vi "Photon Counter Control Panel.vi"(8 "error in (no error)":errorcluster) -> (0 "error out":errorcluster)   [LabVIEW 2015]
uses:
  Public/Typedefs/Gate Mode.ctl
  Public/Typedefs/Discriminator Output.ctl
  <vilib>/express/express shared/transition.llb/Dynamic To Waveform Array.vi
  <vilib>/express/express signal manip/GetorSetDDTAttributes/Set DDT Attributes/SetT0.vi
  <vilib>/express/express shared/transition.llb/Waveform Array To Dynamic.vi
  <vilib>/express/express signal manip/GetorSetDDTAttributes/Set DDT Attributes/Set DDT Properties.xnode
  SR400.lvlib
panel:
  in  "Monitor":bool
  in  "Start Scan":bool caption="Start Monitored Scan"
  in  "Stop Scan":bool
  out "Counter B":dbl(graph)=996.0
  out "Counter A":dbl(graph)=944.0
  out "Scan Start Time":timestamp=timestamp(3611338511.309165 s since 1904-01-01)
  out "Counter A":dbl(graph)=5052.0
  out "Counter B":dbl(graph)=5104.0
  in  "Read Buffer Data":bool
  out "Scan Done":bool
  out "Data Ready":bool
  in  "Query Status Byte":bool
  out "Scan Start Time":timestamp=timestamp(3611333596.390047 s since 1904-01-01)
  out "Filename Out":path=path "C:/Users/physics/Desktop/test_1.xlsx"
  in  "GPIB Address":i32=23 min=0 max=30 step=1
  in  "Stop Unmonitored Scan":bool
  in  "Disc A Mode":T1
  in  "Disc B Mode":T1
  in  "Disc B Slope":enum16{"Rise", "Fall"}(ring)
  in  "Disc A Slope":enum16{"Rise", "Fall"}(ring)
  in  "Trigger Slope":enum16{"Rise", "Fall"}(ring)
  in  "Set Gate Widths":bool
  in  "Set Gate Mode":bool
  out "Actual":dbl[unit]=0.5 caption="Current Dwell Time"
  in  "Target":dbl[unit]=0.5 caption="Dwell Time Target" min=0.0 max=60.0 step=0.5 format="%#_1g"
  in  "Set Dwell Time":bool
  in  "Target":i32=10 caption="Number of Periods Target" min=0 max=2000 step=1
  out "Actual":dbl=10.0 caption="Number of Periods Current"
  in  "Set # Periods":bool
  in  "Scan End Mode":enum16{"Stop", "Start"}(ring)
  in  "Disc B Lvl":dbl=-0.012 format="%#_13g"
  in  "Disc A Lvl":dbl=-0.012 format="%#_13g"
  in  "Display Mode":enum16{"Continuous", "Hold"}(ring)
  in  "Initialize":bool
  in  "Internal / External":bool
  in  "Set Count Time":bool
  in  "Counter B Input":enum16{"10 MHz", "INPUT 1", "INPUT 2", "TRIG"}(ring)=enum."INPUT 1"
  in  "Counter A Input":enum16{"10 MHz", "INPUT 1", "INPUT 2", "TRIG"}(ring)=enum."INPUT 1"
  in  "Count Mode":T2(ring)
  in  "Trigger Level":dbl=1.25 format="%#_13g"
  in  "VISA Resource Name":refnum<visa-resource-name>="GPIB0::23::INSTR"
  in  "Photon Counter SR 400":T3={"Mode"=0, "Count Time"=1.0, "Trigger Frequency"=10000000.0, "Trigger External?"=FALSE, "Gate A Mode"=0, "Gate A Width"=5e-09, "Gate A Delay"=5e-09, "Gate B Mode"=0, "Gate B Width"=5e-09, "Gate B Delay"=5e-09} {"Mode" items=["A,B For T Preset", "A-B For T Preset", "A+B For T Preset", "A For B Preset"]; "Gate A Mode" items=["CW", "Fixed"]; "Gate B Mode" items=["CW", "Fixed"]}
  out "Update visible/hidden":bool
  out "Actual":T4
  out "Actual":T4
  in  "stop":bool
  in  "Read to\nControl":bool
  in  "Read":bool
  out "Actual":dbl=5.0
  out "Actual":dbl=5.0
  in  "Target":dbl=5.0 caption="Gate A Width Percent Target"
  in  "Target":dbl=5.0 caption="Gate A Percent Target"
  in  "Gate Width: Time / Percent":bool caption="Time/Percent"
  in  "Start / Middle":bool
  in  "Target":T4 caption="Gate B Mode Target"
  in  "Target":T4 caption="Gate A Mode Target"
  out "Actual":dbl[unit]=10000000.0 caption="Trigger Freq"
  in  "Target":dbl[unit]=10000000.0 caption="Trigger Freq. Target"
  in  "Set Time & Freq.":bool
  in  "# Triggers vs Freq/Time":bool=TRUE
  out "Actual":dbl=10000000.0 caption="External Trigger # Cycles Current" format="%^#_6g"
  in  "Target":dbl=10000000.0 format="%^#_6g"
  in  "Set # of Triggers":bool
  in  "Target":dbl[unit]=5e-09 caption="Gate B Width Target"
  in  "Target":dbl[unit]=5e-09 caption="Gate A Width Target"
  out "Actual":dbl[unit]=5e-09 format="%^#_6g"
  out "Actual":dbl[unit]=5e-09 format="%^#_6g"
  out "Actual":dbl[unit]=5e-09
  out "Actual":dbl[unit]=5e-09
  in  "Target":dbl[unit]=5e-09
  in  "Target":dbl[unit]=5e-09 caption="Gate A Delay Target"
  in  "Set Gate Delays":bool
  in  "Start Unmonitored Scan":bool
  in  "Target":dbl[unit]=1.0 caption="Count Time Target" min=0.0 step=0.5 format="%#_1f"
  out "Actual":dbl[unit]=1.0 caption="Count Time Current" min=0.0 max=10000.0 step=1.0 format="%#_7g"
  # "Gates"
  # "Setup"
  # "Acquisition"
  # "Gate B Mode"
  # "Gate A Mode"
  # "# of Periods"
  # "Count Time"
  # "Gate A Width"
  # "Gate B Width"
  # "Dwell Time"
  # "Gate A Delay"
  # "Gate B Delay"
  # "Set values and initialize.\n\nSettings you can \"live\" update w/o initialization:\n        All Gate Params\n        Count Time (Only largest sig digit used)\n        Dwell Time (Only largest sig digit used)\n        External Trigger\n        # Periods\n\nSettings without a \"Set _____\" button need to be changed by initialization.\n\nAll variables are initialized, but \"live\" params do not show current value until you press the set button for that parameter.\n\n\"Read\" sets the \"Current\" indicators to what the hardware has set.\n\n\"Read to Control\" sets the \"Setpoint\" controls to the values from \"Read\""
  # "Discriminator/Trigger"
  # "Do not save data until after the scan is done or stopped.\n\nMonitored data may be erroneous due to communication delay\n\nTimestamps are relative to saving the data, not when data was taken. Datapoints need a reference (included scan start time)."
  # "External Trigger # of Cycles/Freq"
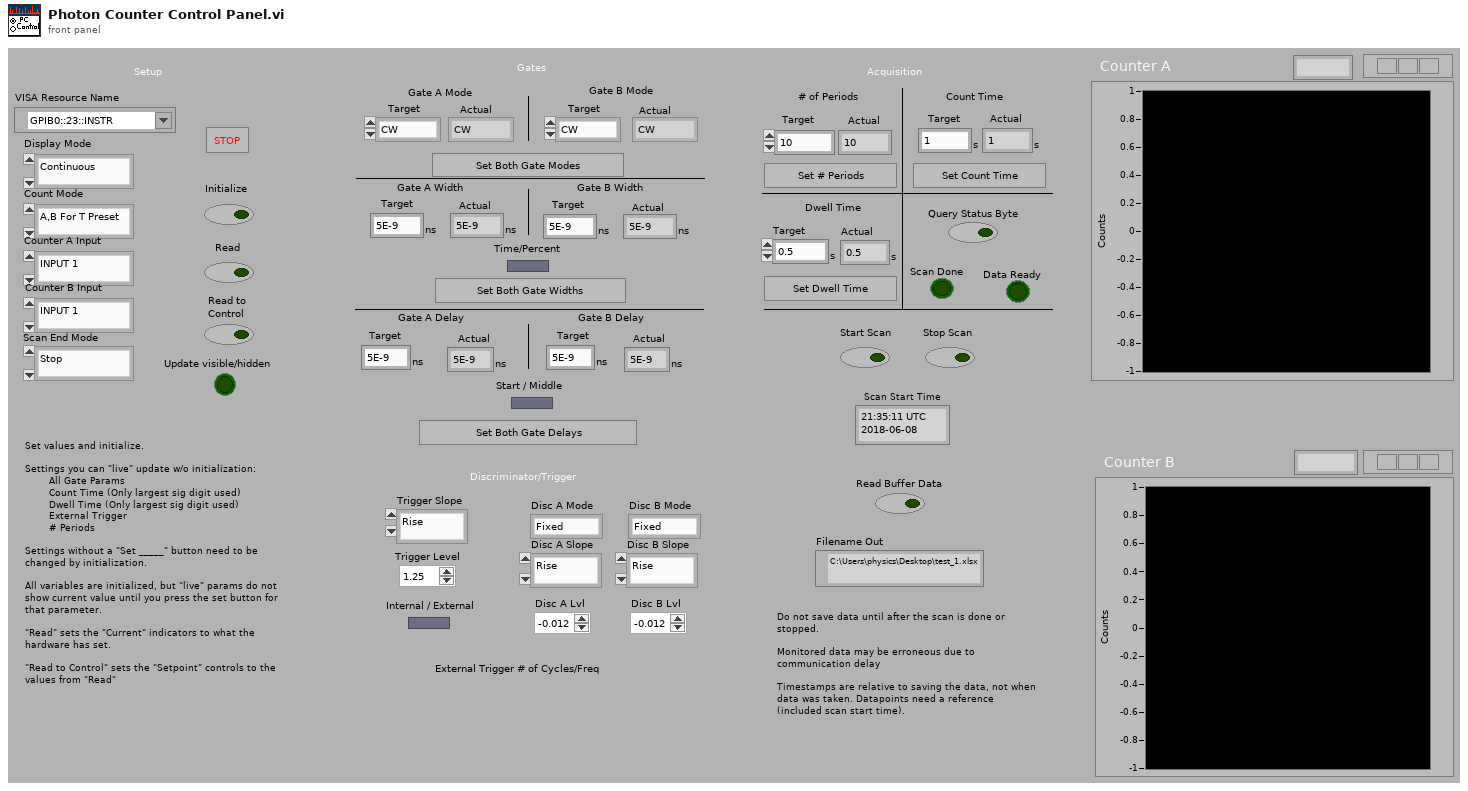
[diagram p1: front panel]
types:
  T1 = typedef "SR400.lvlib/Discriminator Output.ctl" = enum16{"Fixed", "Scan"}
  T2 = enum16{"A,B For T Preset", "A-B For T Preset", "A+B For T Preset", "A For B Preset"}
  T3 = cluster{"Mode":u16, "Count Time":dbl[unit], "Trigger Frequency":dbl[unit], "Trigger External?":bool, "Gate A Mode":u16, "Gate A Width":dbl[unit], "Gate A Delay":dbl[unit], "Gate B Mode":u16, "Gate B Width":dbl[unit], "Gate B Delay":dbl[unit]}
  T4 = typedef "SR400.lvlib/Gate Mode.ctl" = enum16{"CW", "Fixed", "Scan"}
  T5 = cluster{"Parameter Changed from front panel":bool, "Data Ready":bool, "Scan Finished":bool, "Counter Overrun":bool, "Rate Error":bool, "Recall Error":bool, "Service Request":bool, "Command Error":bool, "Triggered":bool, "Inhibited":bool, "Counting":bool}
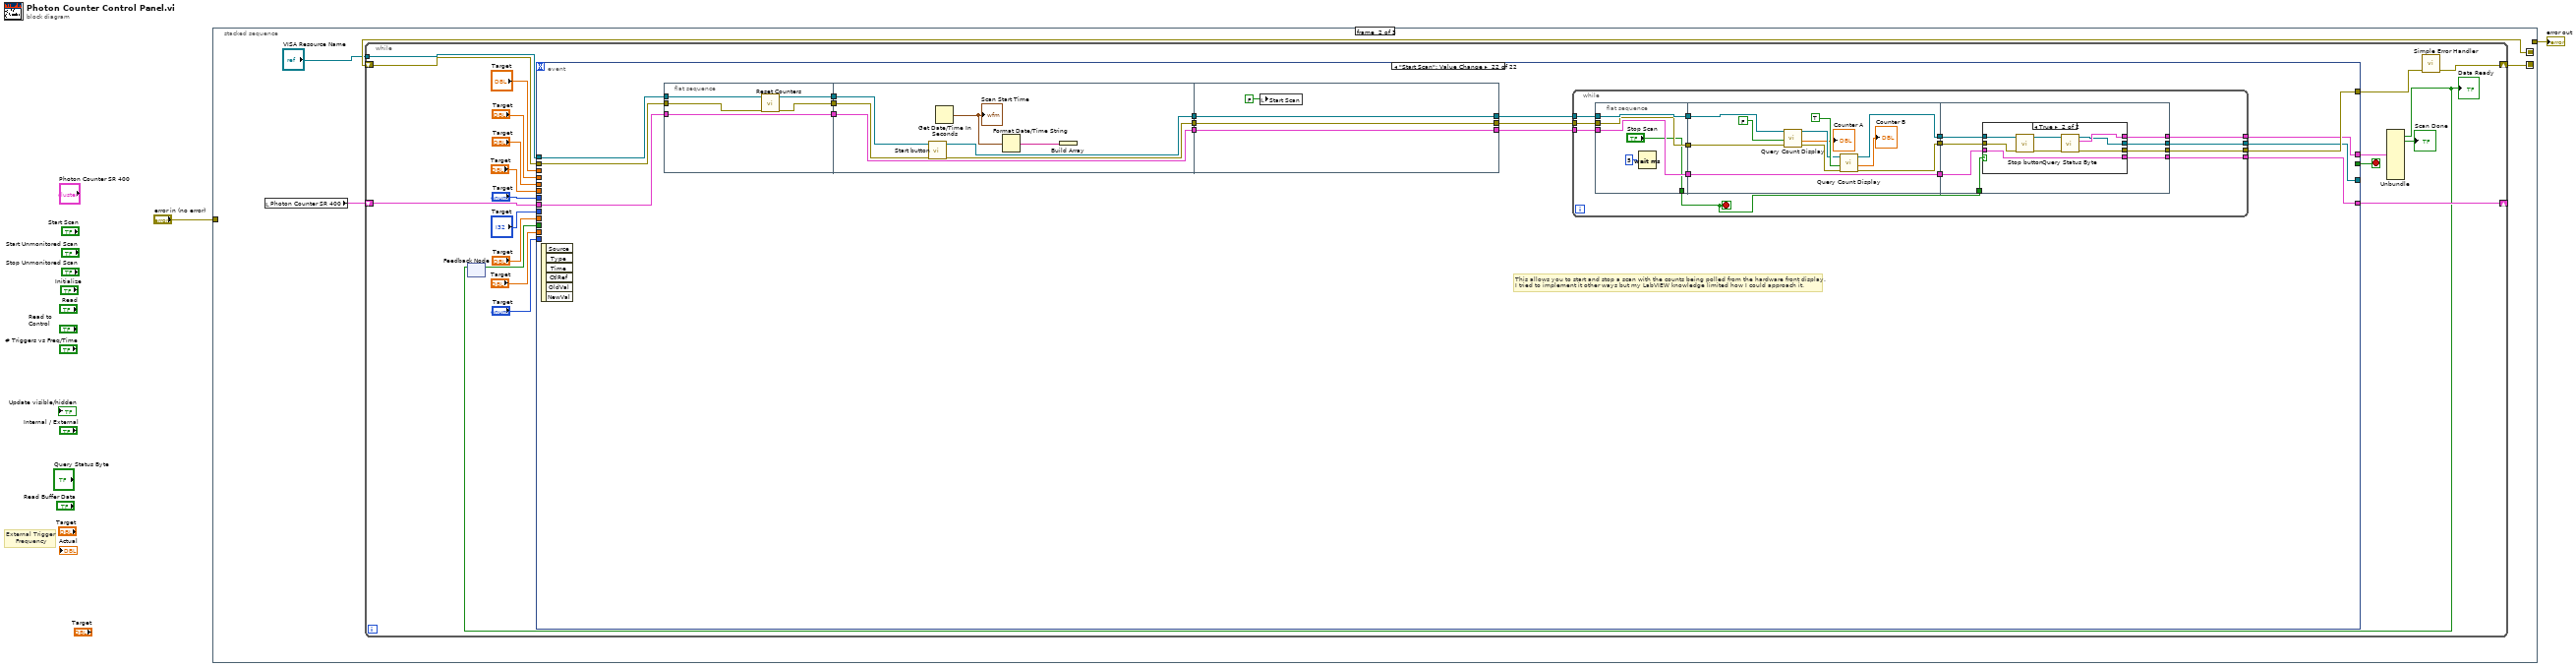
[diagram p0: block diagram]
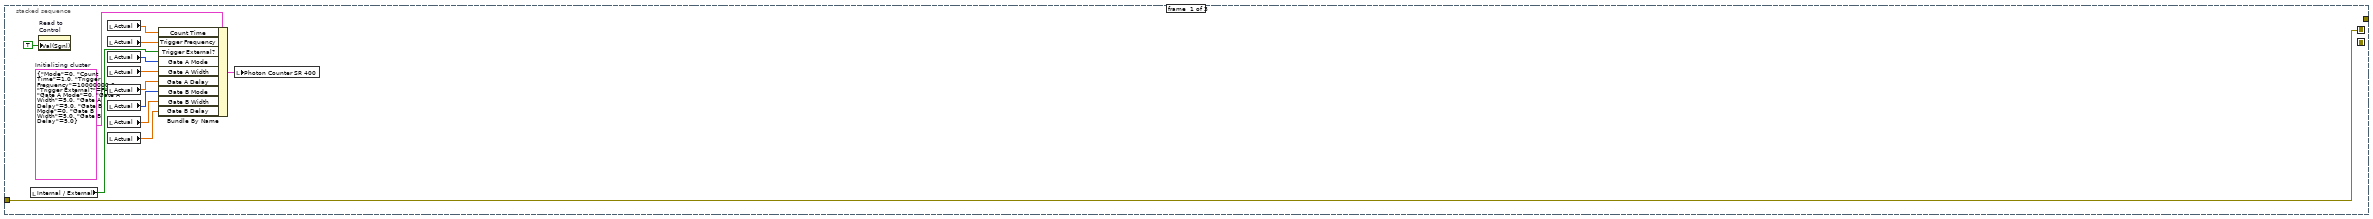
[diagram p2: hidden frame]
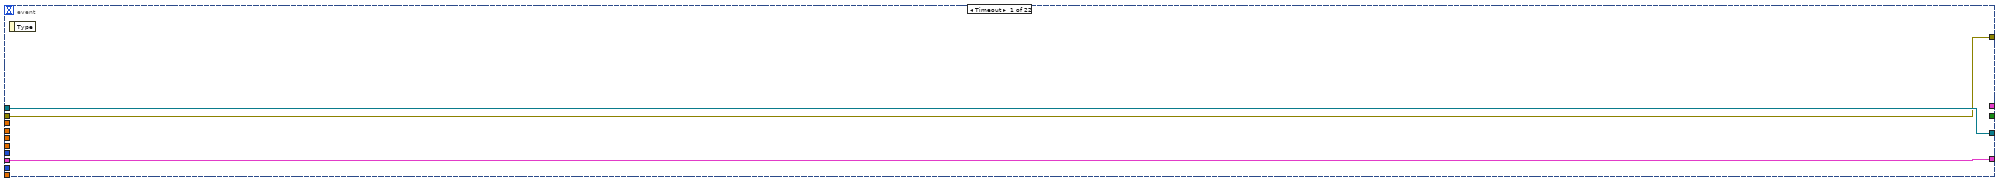
[diagram p3: hidden frame]
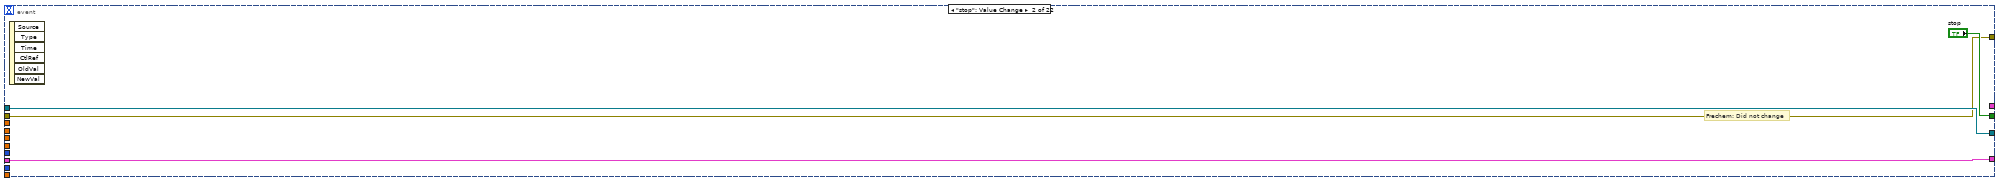
[diagram p4: hidden frame]
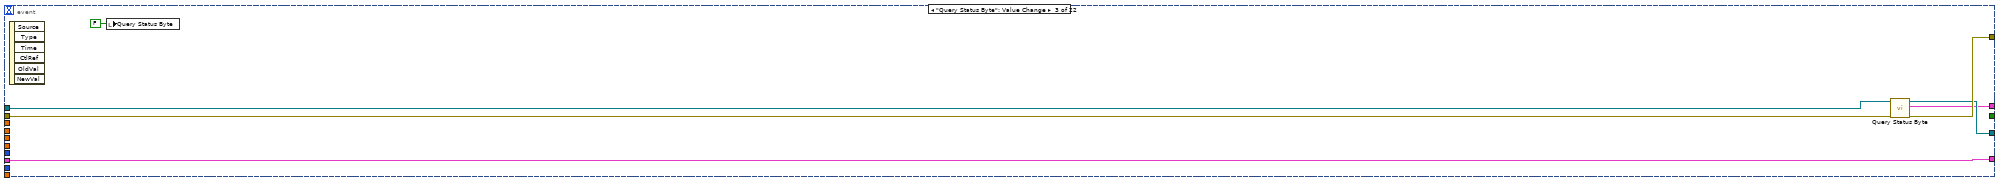
[diagram p5: hidden frame]
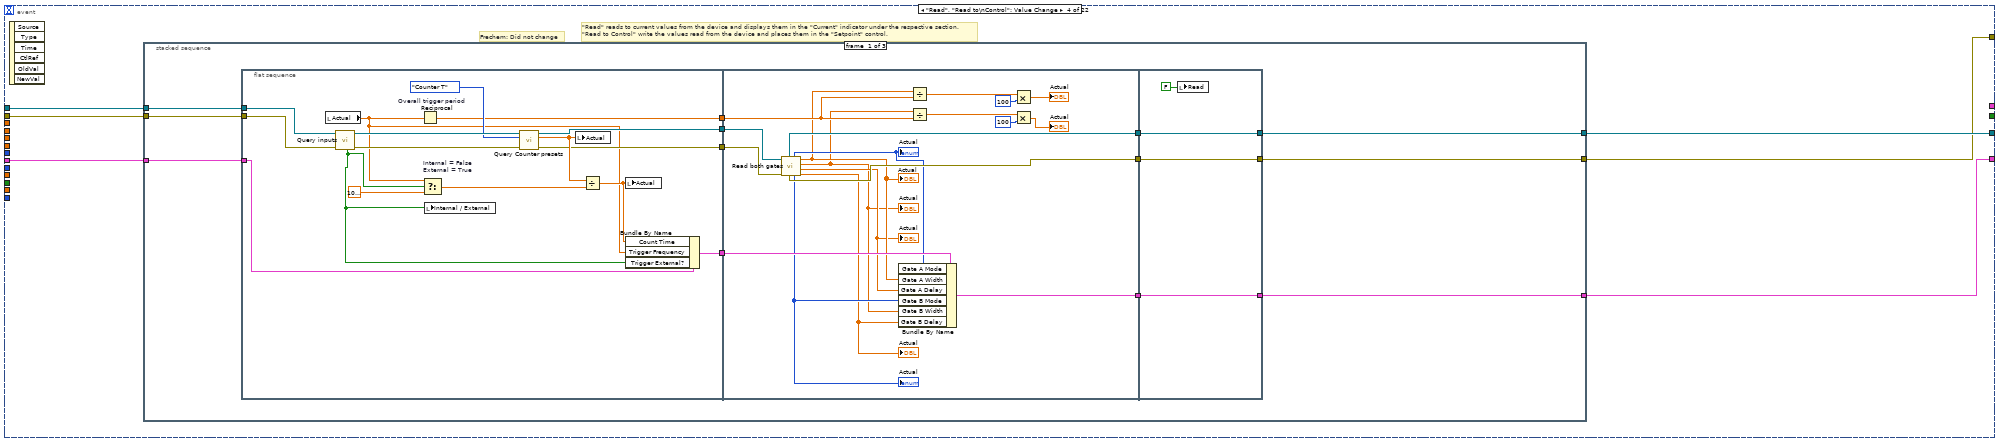
[diagram p6: hidden frame]
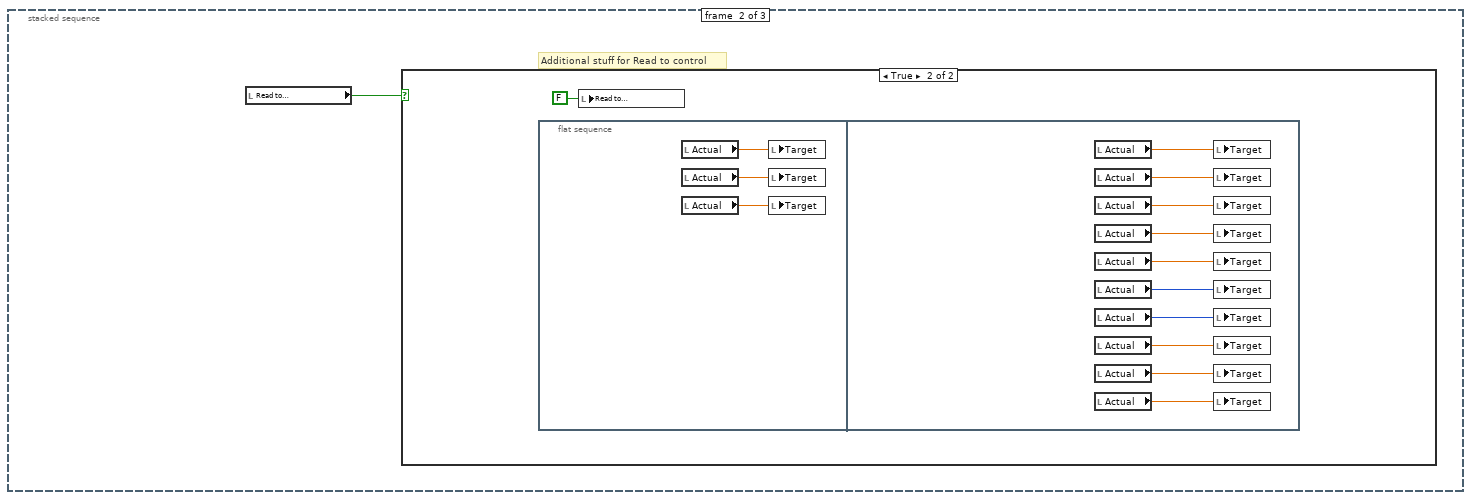
[diagram p7: hidden frame]
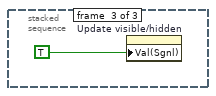
[diagram p9: hidden frame]
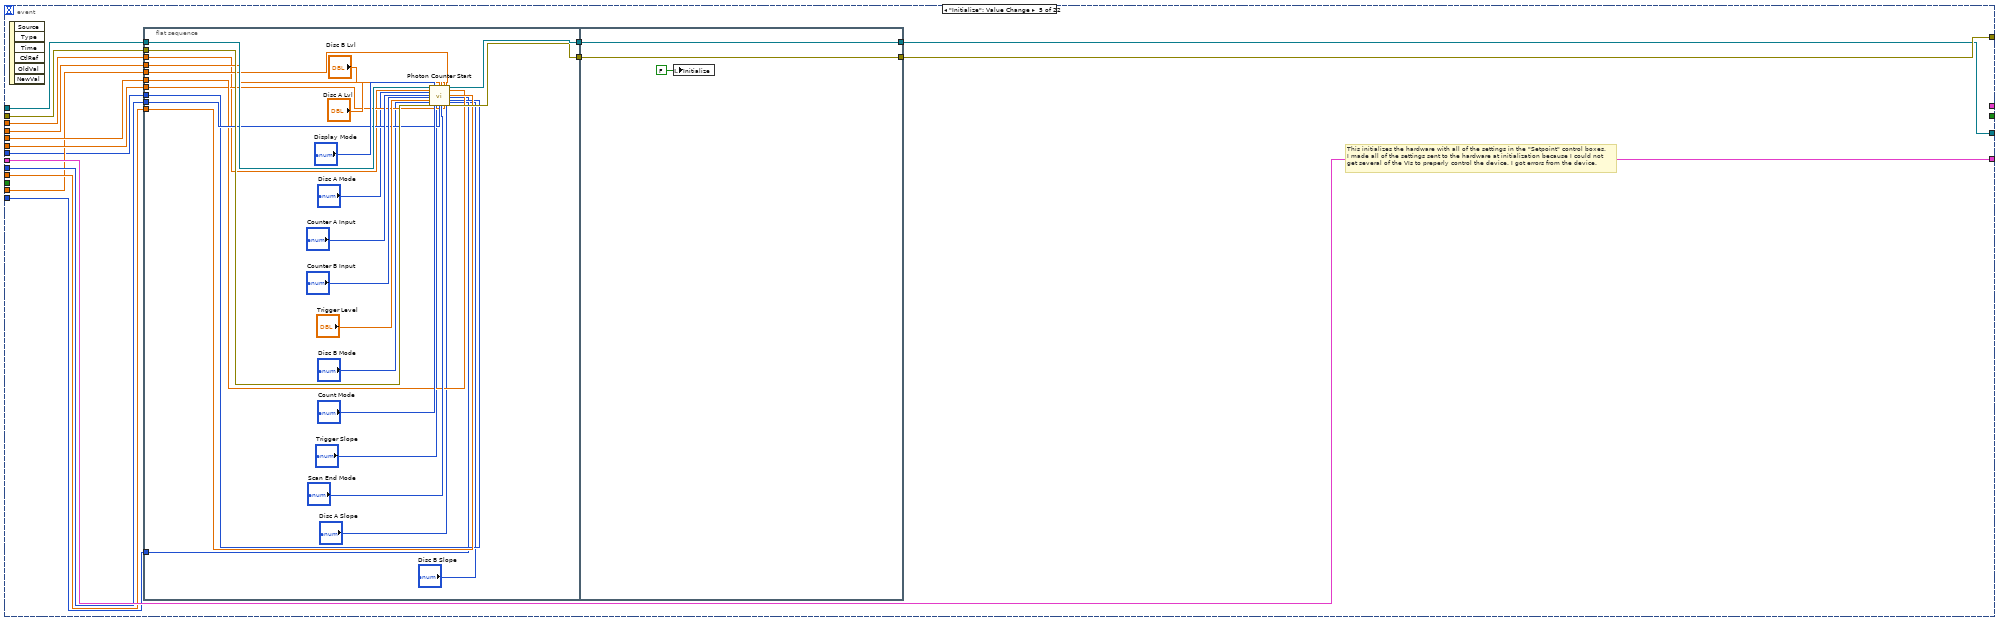
[diagram p10: hidden frame]
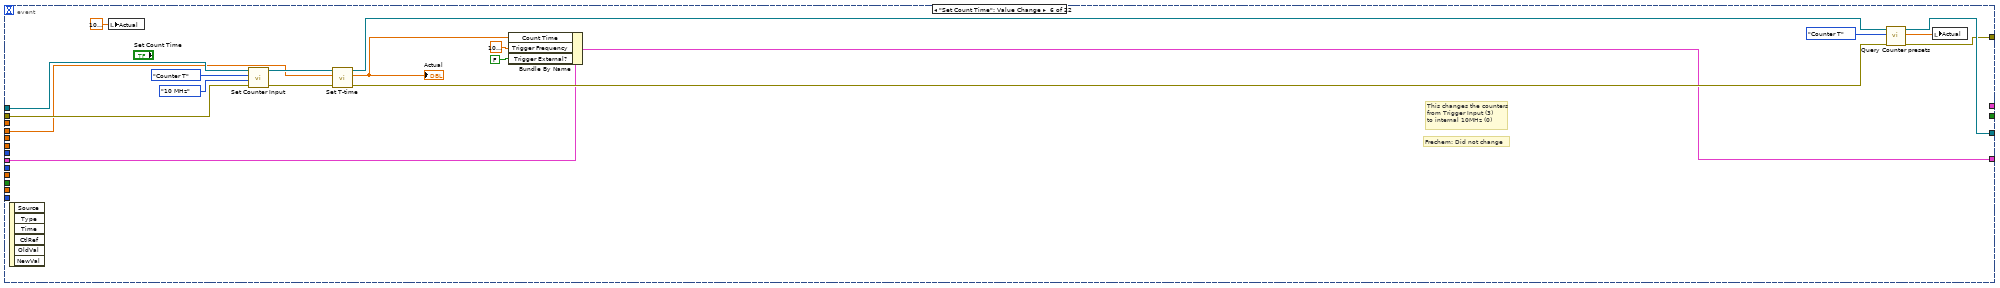
[diagram p11: hidden frame]
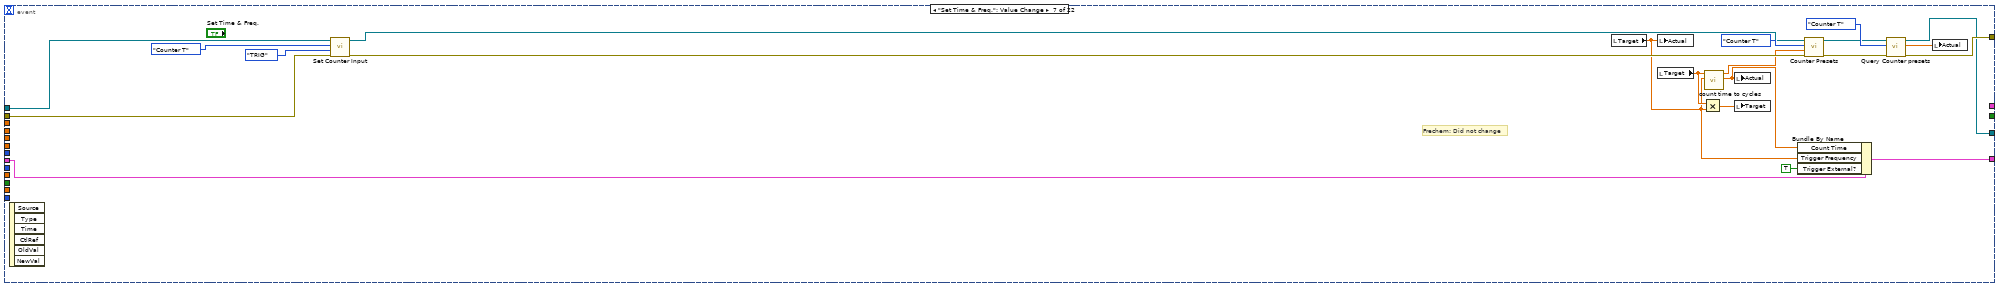
[diagram p12: hidden frame]
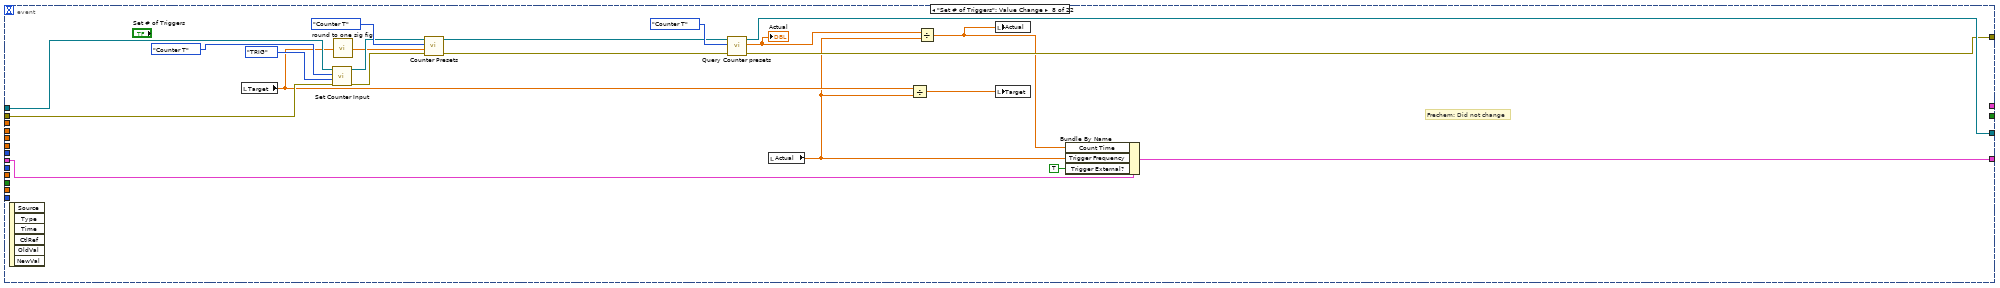
[diagram p13: hidden frame]
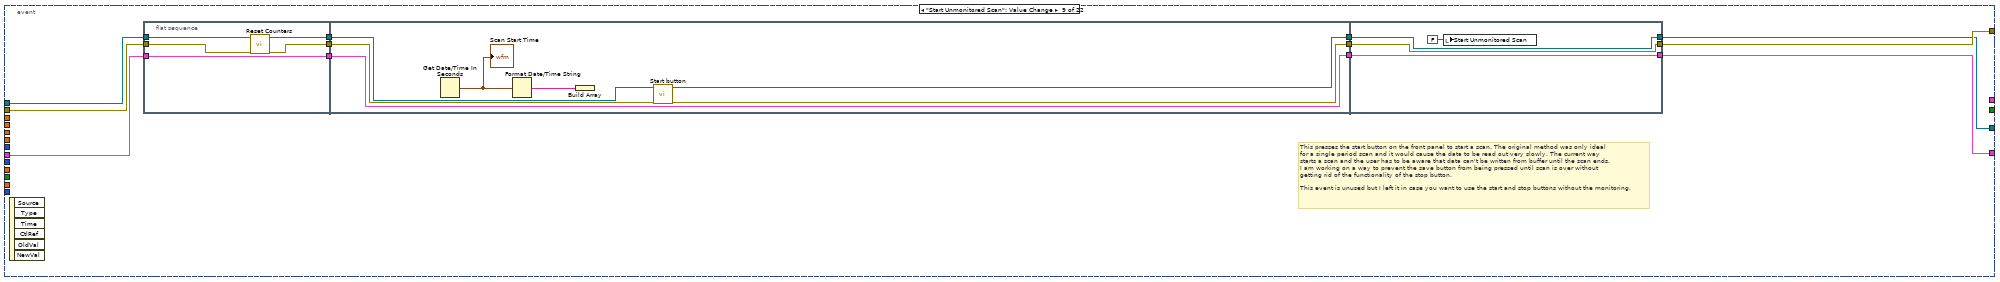
[diagram p14: hidden frame]
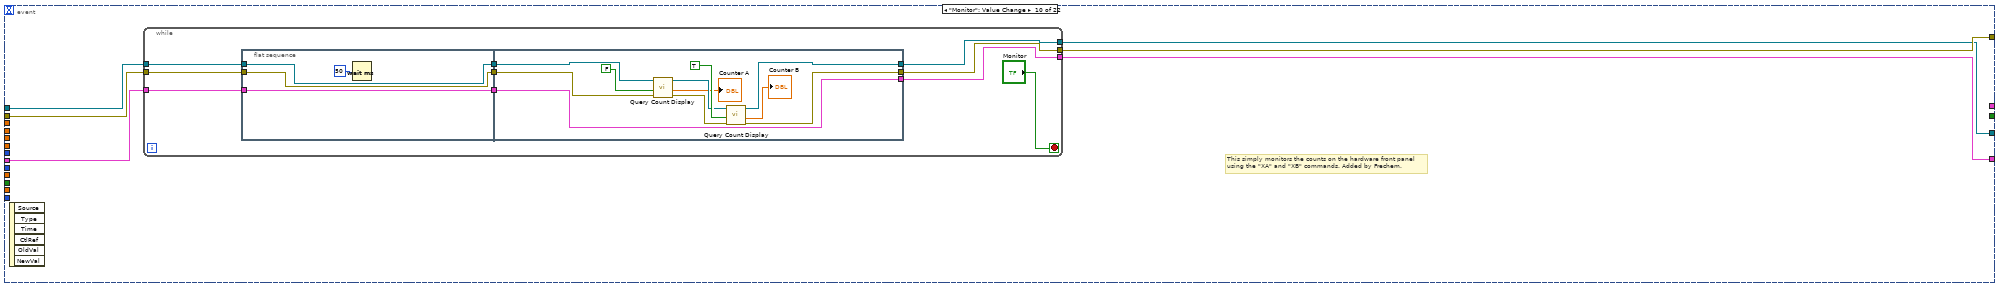
[diagram p15: hidden frame]
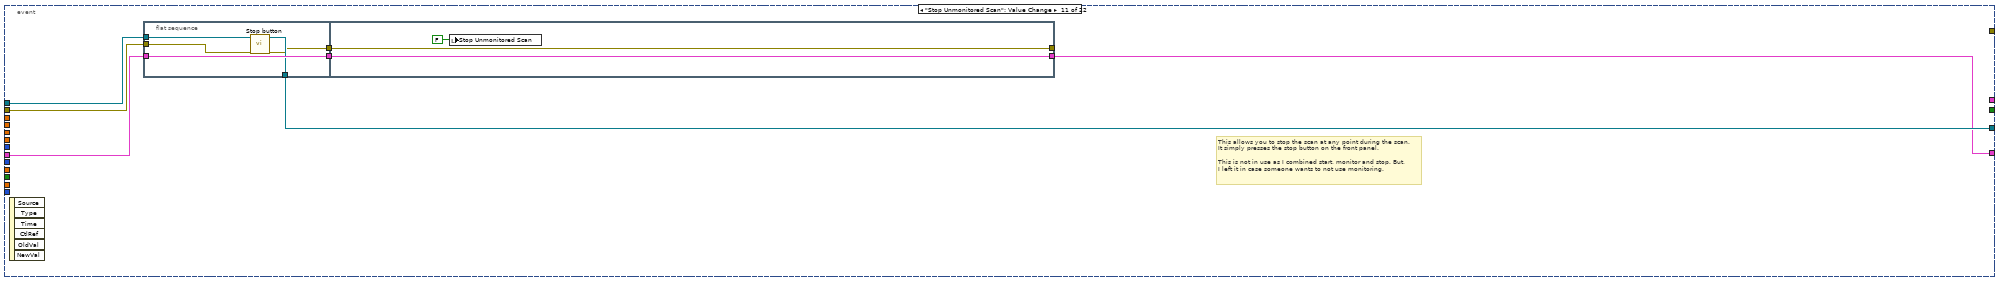
[diagram p16: hidden frame]
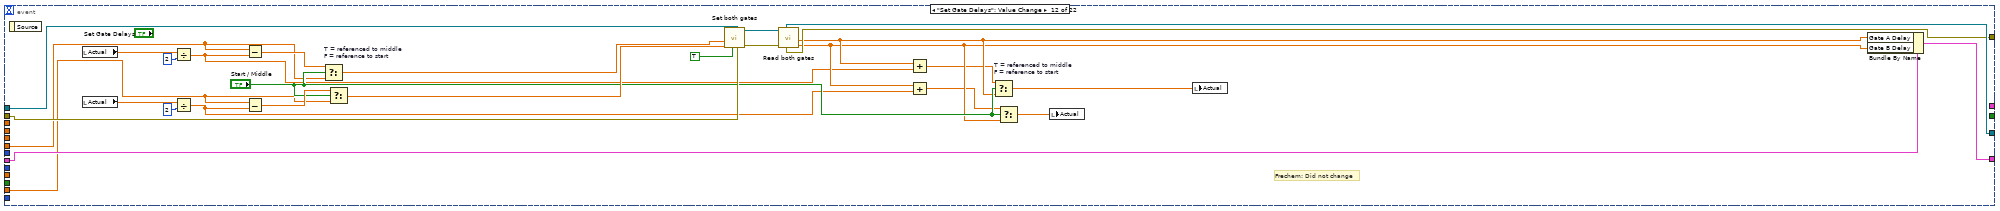
[diagram p17: hidden frame]
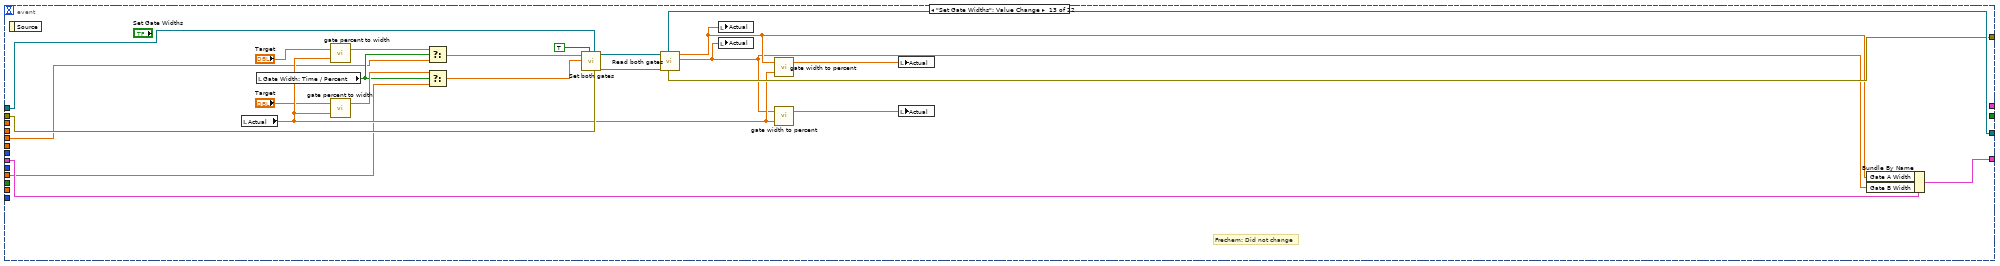
[diagram p18: hidden frame]
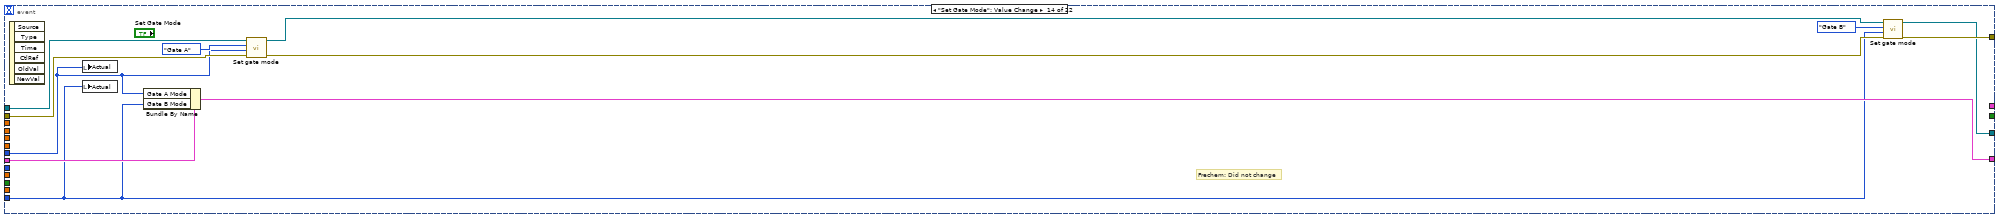
[diagram p19: hidden frame]
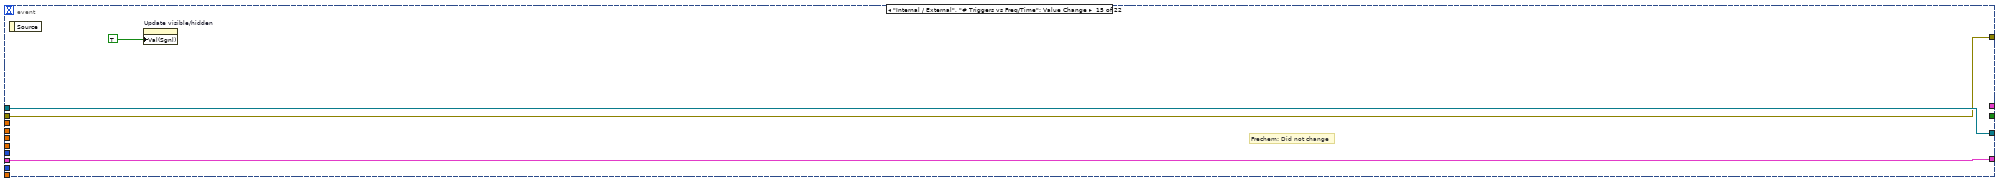
[diagram p20: hidden frame]
diagram:
  # "External Trigger \n     Frequency"
  n1 = stacked-sequence {
    seq-local: [w5 _ _] -> [_ w19 _]
    seq-local: [_ w18 _] -> [_ _ w655]
    tunnel: "error in (no error)" -> [w5 _ _]
    tunnel: [_ _ w655] -> w2
    frame #0 {
      w3 = T3 {"Mode"=0, "Count Time"=1.0, "Trigger Frequency"=10000000.0, "Trigger External?"=FALSE, "Gate A Mode"=0, "Gate A Width"=5.0, "Gate A Delay"=5.0, "Gate B Mode"=0, "Gate B Width"=5.0, "Gate B Delay"=5.0}  # Initializing cluster
      n2 = local read "Internal / External"() -> (w12:bool)
      n3 = property on="Read to\nControl" class="Bool (strict)"("Val(Sgnl)"=TRUE ("Value (Signaling)")) -> ()  [unwired: 2 in, 2 out]
      n4 = local read "Actual"() -> (w14:dbl[unit])
      n5 = local read "Actual"() -> (w13:dbl[unit])
      n6 = local read "Actual"() -> (w11:T4)
      n7 = local read "Actual"() -> (w10:dbl[unit])
      n8 = local read "Actual"() -> (w9:dbl[unit])
      n9 = local read "Actual"() -> (w6:T4)
      n10 = local read "Actual"() -> (w7:dbl[unit])
      n11 = local read "Actual"() -> (w8:dbl[unit])
      n12 = Bundle By Name(cluster=w3, "Count Time"=w14, "Trigger Frequency"=w13, "Trigger External?"=w12, "Gate A Mode"=w11, "Gate A Width"=w10, "Gate A Delay"=w9, "Gate B Mode"=w6, "Gate B Width"=w7, "Gate B Delay"=w8) -> (w4:T3)
      n13 = local write "Photon Counter SR 400"(w4) -> ()
    }
    frame #1 {
      n14 = local read "Photon Counter SR 400"() -> (w17:T3)
      n15 = while {
        shift-right: [w36] -> _
        shift-left: w17 -> [w35]
        shift-right: [w38] -> w18
        shift-left: w19 -> [w22]
        tunnel: "VISA Resource Name" -> [w21]
        stop <- w37 stop-if-true
        n16 = feedback #1() -> (w23:bool)  [unwired: 1 in]
        n17 = event shown="[21] \"Start Scan\": Value Change" {
          selector: _ -> [_ _ _ _ _ _ _ _ _ _ _ _ _ _ _ _ _ _ _ _ _ _]
          dyn-events: _ -> [_ _ _ _ _ _ _ _ _ _ _ _ _ _ _ _ _ _ _ _ _ _]
          timeout: _ -> [_ _ _ _ _ _ _ _ _ _ _ _ _ _ _ _ _ _ _ _ _ _]
          tunnel: [w41 w44 w48 w57 w139 w189 w207 w231 w241 w266 w294 w321 w353 w363 w374 w377 w403 w436 w452 w459 w480 w572] -> _
          tunnel: w22 -> [w40 w43 w50 w59 w143 w180 w201 w223 w245 w265 w297 w335 w354 w367 w373 w375 w402 w435 w449 w465 w483 w575]
          tunnel: [w40 w43 w49 w56 w142 w188 w208 w230 w243 w267 _ w319 w352 w364 w373 w376 w402 w435 w451 w458 w482 w574] -> w39
          tunnel: w21 -> [w41 w44 w51 w58 w137 w181 w202 w224 w237 w264 w296 w334 w355 w368 w374 w377 w403 w436 w450 w466 w481 w576]
          tunnel: w35 -> [w42 w45 w53 w55 w138 w178 w196 w217 w239 w263 w295 w333 w341 w362 w372 w378 w404 w434 w448 w457 w479 w577]
          tunnel: [w42 w45 w53 w54 w138 w177 w195 w216 w238 w262 w293 w332 w340 w361 w372 w378 w404 w434 w448 w457 w478 w573] -> w36
          tunnel: [_ "stop" _ _ _ _ _ _ _ _ _ _ _ _ _ _ _ _ _ _ _ _] -> w37
          tunnel: "Target" -> [_ _ _ _ w136 _ _ _ _ _ _ _ _ _ _ _ _ _ w447 _ w477 _]
          tunnel: "Target" -> [_ _ _ _ w135 _ _ _ _ _ _ _ w337 _ _ _ _ _ _ _ _ _]
          tunnel: "Target" -> [_ _ _ _ w134 _ _ _ _ _ _ _ w336 _ _ _ _ _ _ _ _ _]
          tunnel: "Target" -> [_ _ _ _ w133 _ _ _ _ _ _ w309 _ _ _ _ _ _ _ _ _ _]
          tunnel: "Target" -> [_ _ _ _ w132 _ _ _ _ _ _ w308 _ _ _ _ _ _ _ _ _ _]
          tunnel: "Target" -> [_ _ _ _ w131 w173 _ _ _ _ _ _ _ _ _ _ _ _ _ _ _ _]
          tunnel: "Target" -> [_ _ _ _ w129 _ _ _ _ _ _ _ _ w360 _ _ _ _ _ _ _ _]
          tunnel: "Target" -> [_ _ _ _ w130 _ _ _ _ _ _ _ _ w359 _ _ _ _ _ _ _ _]
          tunnel: "Target" -> [_ _ _ _ w128 _ _ _ _ _ _ _ _ _ _ _ _ _ _ w463 _ _]
          tunnel: [_ _ w47 _ _ _ _ _ _ _ _ _ _ _ _ _ _ _ _ _ w471 w571] -> w25
          tunnel: w23 -> [_ _ _ _ _ _ _ _ _ _ _ _ _ _ _ _ _ _ _ _ w476 _]
          event Timeout {
            n18 = event-data() -> ()  [unwired: 2 out]
          }
          event "stop": Value Change {
            # "Frechem: Did not change"
            n19 = event-data() -> ()  [unwired: 7 out]
          }
          event "Query Status Byte": Value Change {
            n20 = event-data() -> ()  [unwired: 7 out]
            n21 = local write "Query Status Byte"(FALSE ("Read Channels")) -> ()
            n22 = call "Query Status Byte.vi"("error in (no error)"=w50, "VISA resource name"=w51) -> ("error out"=w49:errorcluster, "Status Register"=w47:T5, "VISA resource name out"=w48:refnum<visa-resource-name>)  [unwired: 7 in]
          }
          event "Read", "Read to\nControl": Value Change {
            # "Frechem: Did not change"
            # "\"Read\" reads to current values from the device and displays them in the \"Current\" indicator under the respective section.\n\"Read to Control\" write the values read from the device and places them in the \"Setpoint\" control."
            n23 = event-data() -> ()  [unwired: 7 out]
            n24 = stacked-sequence {
              tunnel: w59 -> [w71 _ _]
              tunnel: w58 -> [w72 _ _]
              tunnel: [w67 _ _] -> w57
              tunnel: [w65 _ _] -> w56
              tunnel: w55 -> [w63 _ _]
              tunnel: [w61 _ _] -> w54
              frame #0 {
                n25 = flat-sequence {
                  tunnel: w72 -> [w88]
                  tunnel: w71 -> [w85]
                  tunnel: [w81] -> w70
                  tunnel: [w80] -> w69
                  tunnel: [w79] -> w68
                  tunnel: w63 -> [w77]
                  tunnel: [w73] -> w62
                  tunnel: w70 -> [w101]
                  tunnel: w69 -> [w100]
                  tunnel: w68 -> [w99]
                  tunnel: [w98] -> w66
                  tunnel: [w97] -> w64
                  tunnel: w62 -> [w96]
                  tunnel: [w89] -> w60
                  tunnel: [w110] -> w67
                  tunnel: w66 -> [w110]
                  tunnel: [w109] -> w65
                  tunnel: w64 -> [w109]
                  tunnel: [w108] -> w61
                  tunnel: w60 -> [w108]
                  frame #0 {
                    n26 = local read "Actual"() -> (w74:dbl[unit])
                    n27 = call "Query inputs.vi"("error in (no error)"=w85, "VISA resource name"=w88) -> ("error out"=w86:errorcluster, "VISA resource name out"=w87:refnum<visa-resource-name>, "Externally-triggered?"=w76:bool)  [unwired: 7 out]
                    n28 = Reciprocal "Overall trigger period"(x=w74) -> (1/x=w79:dbl[unit])
                    n29 = Select "Internal = False\nExternal = True"(t=w74, s=w76, f=dbl[unit] 10000000.0 ("freq")) -> (s? t:f=w83:dbl[unit])
                    n30 = local write "Internal / External"(w76) -> ()
                    n31 = call "Query Counter presets.vi"("error in (no error)"=w86, "Counter (Def: T)"=enum16{"Invalid", "Counter B", "Counter T"}."Counter T" ("i (0)"), "VISA resource name"=w87) -> ("error out"=w80:errorcluster, "Number of triggers"=w82:dbl, "VISA resource name out"=w81:refnum<visa-resource-name>)  [unwired: 6 out]
                    n32 = local write "Actual"(w82) -> ()
                    n33 = Divide(x=w82, y=w83) -> (x/y=w75:dbl[unit])
                    n34 = local write "Actual"(w75) -> ()
                    n35 = Bundle By Name(cluster=w77, "Count Time"=w75, "Trigger Frequency"=w74, "Trigger External?"=w76) -> (w73:T3)
                  }
                  frame #1 {
                    n36 = call "Read both gates.vi"("error in (no error)"=w100, "VISA resource name"=w101) -> ("Gate B Delay"=w90:dbl[unit], "Gate A Delay"=w93:dbl[unit], "Gate B Width"=w91:dbl[unit], "Gate A Width"=w94:dbl[unit], "Current mode B"=w92:enum16{"CW", "Fixed", "Scan"}, "Current mode A"=w95:enum16{"CW", "Fixed", "Scan"}, "error out"=w97:errorcluster, "VISA resource name out"=w98:refnum<visa-resource-name>)  [unwired: 2 out]
                    "Actual" <- w91
                    "Actual" <- w94
                    "Actual" <- w93
                    "Actual" <- w90
                    "Actual" <- w95
                    "Actual" <- w92
                    n37 = Bundle By Name(cluster=w96, "Gate A Mode"=w95, "Gate A Width"=w94, "Gate A Delay"=w93, "Gate B Mode"=w92, "Gate B Width"=w91, "Gate B Delay"=w90) -> (w89:T3)
                    n38 = Divide(x=w94, y=w99) -> (x/y=w103:dbl)
                    n39 = Divide(x=w91, y=w99) -> (x/y=w105:dbl)
                    n40 = Multiply(x=w103, y=i8 100) -> (x*y=→"Actual":dbl)
                    n41 = Multiply(x=w105, y=i8 100) -> (x*y=→"Actual":dbl)
                  }
                  frame #2 {
                    n42 = local write "Read"(FALSE ("Read")) -> ()
                  }
                }
              }
              frame #1 {
                # "Additional stuff for Read to control"
                n43 = local read "Read to\nControl"() -> (w112:bool)
                n44 = case shown="True" w112 {
                  frame False {
                  }
                  frame True {
                    n45 = flat-sequence {
                      frame #0 {
                        n46 = local read "Actual"() -> (w116:dbl[unit])
                        n47 = local read "Actual"() -> (w114:dbl[unit])
                        n48 = local read "Actual"() -> (w115:dbl)
                        n49 = local write "Target"(w116) -> ()
                        n50 = local write "Target"(w114) -> ()
                        n51 = local write "Target"(w115) -> ()
                      }
                      frame #1 {
                        n52 = local read "Actual"() -> (w117:dbl[unit])
                        n53 = local read "Actual"() -> (w126:dbl[unit])
                        n54 = local read "Actual"() -> (w122:dbl[unit])
                        n55 = local read "Actual"() -> (w125:dbl)
                        n56 = local read "Actual"() -> (w124:dbl[unit])
                        n57 = local read "Actual"() -> (w120:T4)
                        n58 = local read "Actual"() -> (w121:T4)
                        n59 = local read "Actual"() -> (w119:dbl[unit])
                        n60 = local read "Actual"() -> (w123:dbl)
                        n61 = local read "Actual"() -> (w118:dbl[unit])
                        n62 = local write "Target"(w117) -> ()
                        n63 = local write "Target"(w126) -> ()
                        n64 = local write "Target"(w122) -> ()
                        n65 = local write "Target"(w125) -> ()
                        n66 = local write "Target"(w124) -> ()
                        n67 = local write "Target"(w120) -> ()
                        n68 = local write "Target"(w121) -> ()
                        n69 = local write "Target"(w119) -> ()
                        n70 = local write "Target"(w123) -> ()
                        n71 = local write "Target"(w118) -> ()
                      }
                    }
                    n72 = local write "Read to\nControl"(FALSE ("Read to Control")) -> ()
                  }
                }
              }
              frame #2 {
                n73 = property on="Update visible/hidden" class="Bool (strict)"("Val(Sgnl)"=TRUE ("Value (Signaling)")) -> ()  [unwired: 2 in, 2 out]
              }
            }
          }
          event "Initialize": Value Change {
            # "This initializes the hardware with all of the settings in the \"Setpoint\" control boxes.\nI made all of the settings sent to the hardware at initialization because I could not \nget several of the VIs to preperly control the device. I got errors from the device."
            n74 = event-data() -> ()  [unwired: 7 out]
            n75 = flat-sequence {
              tunnel: w143 -> [w169]
              tunnel: [w168] -> w141
              tunnel: [w167] -> w140
              tunnel: w137 -> [w166]
              tunnel: w136 -> [w157]
              tunnel: w135 -> [w156]
              tunnel: w134 -> [w155]
              tunnel: w133 -> [w154]
              tunnel: w132 -> [w153]
              tunnel: w131 -> [w152]
              tunnel: w130 -> [w151]
              tunnel: w129 -> [w150]
              tunnel: w128 -> [w149]
              tunnel: [w171] -> w142
              tunnel: [w172] -> w139
              tunnel: w141 -> [w172]
              tunnel: w140 -> [w171]
              frame #0 {
                n76 = call "Photon Counter Start.vi"("VISA resource name"=w166, "Dwell Time"=w149, "Disc A Mode"="Disc A Mode", "Count A Input"="Counter A Input", "Count B Input"="Counter B Input", "Trigger Level"="Trigger Level", "Disc B Mode"="Disc B Mode", "errorIN"=w169, "Display Mode"="Display Mode", "Count Mode"="Count Mode", "Trigger Slope"="Trigger Slope", "Disc A Lvl"="Disc A Lvl", "# of periods"=w157, "Disc B Lvl"="Disc B Lvl", "Scan End Mode"="Scan End Mode", "Count Time Set"=w152, "Gate A Delay (def: 0 s)"=w154, "Gate B Delay (def: 0 s)"=w153, "Disc A\nSlope"="Disc A Slope", "Gate A Width (def: 0 s)"=w155, "Gate B Width (def: 0 s)"=w156, "Gate B Mode"=w150, "Gate A Mode"=w151, "Disc B\nSlope"="Disc B Slope") -> ("VISA resource name out"=w168:refnum<visa-resource-name>, "errorOUT"=w167:errorcluster)  [unwired: 2 in]
              }
              frame #1 {
                n77 = local write "Initialize"(FALSE ("Re-initialize")) -> ()
              }
            }
          }
          event "Set Count Time": Value Change {
            # "Frechem: Did not change"
            # "This changes the counters\nfrom Trigger Input (3)\nto internal 10MHz (0)"
            n78 = event-data() -> ()  [unwired: 7 out]
            n79 = local write "Actual"(dbl[unit] 10000000.0 ("freq")) -> ()
            n80 = call "Set Counter Input.vi"("error in (no error)"=w180, "Input (def: 10 MHz)"=enum16{"10 MHz", "INPUT 1", "INPUT 2", "TRIG"}."10 MHz" ("n (0.000000)"), "Counter (def: A)"=enum16{"Counter A", "Counter B", "Counter T"}."Counter T" ("i (0) 2"), "VISA resource name"=w181) -> ("error out"=w183:errorcluster, "VISA resource name out"=w182:refnum<visa-resource-name>)  [unwired: 6 out]
            n81 = call "Set T-time.vi"("errorIN"=w183, "Count Time Set"=w173, "VISA resource name"=w182) -> ("errorOUT"=w184:errorcluster, "ttimeOUT"=w176:dbl[unit], "VISA resource name out"=w187:refnum<visa-resource-name>)  [unwired: 4 out]
            "Actual" <- w176
            n82 = Bundle By Name(cluster=w178, "Count Time"=w176, "Trigger Frequency"=dbl[unit] 10000000.0, "Trigger External?"=FALSE) -> (w177:T3)
            n83 = call "Query Counter presets.vi"("error in (no error)"=w184, "Counter (Def: T)"=enum16{"Invalid", "Counter B", "Counter T"}."Counter T" ("i (0)"), "VISA resource name"=w187) -> ("error out"=w188:errorcluster, "Number of triggers"=w190:dbl, "VISA resource name out"=w189:refnum<visa-resource-name>)  [unwired: 6 out]
            n84 = local write "Actual"(w190) -> ()
          }
          event "Set Time & Freq.": Value Change {
            # "Frechem: Did not change"
            n85 = event-data() -> ()  [unwired: 7 out]
            n86 = call "Set Counter Input.vi"("error in (no error)"=w201, "Input (def: 10 MHz)"=enum16{"10 MHz", "INPUT 1", "INPUT 2", "TRIG"}."TRIG" ("n (0.000000)"), "Counter (def: A)"=enum16{"Counter A", "Counter B", "Counter T"}."Counter T" ("i (0) 2"), "VISA resource name"=w202) -> ("error out"=w203:errorcluster, "VISA resource name out"=w204:refnum<visa-resource-name>)  [unwired: 6 out]
            n87 = local read "Target"() -> (w192:dbl[unit])
            n88 = local write "Actual"(w192) -> ()
            n89 = local read "Target"() -> (w197:dbl[unit])
            n90 = Multiply(x=w197, y=w192) -> (x*y=w198:dbl)
            n91 = call "count time to cycles.vi"("Trigger Freq"=w192, "Count Time Set"=w197) -> ("Count Time Current"=w193:dbl[unit], "Number of triggers"=w199:dbl)  [unwired: 3 in, 1 out]
            n92 = local write "Actual"(w193) -> ()
            n93 = local write "Target"(w198) -> ()
            n94 = Bundle By Name(cluster=w196, "Count Time"=w193, "Trigger Frequency"=w192, "Trigger External?"=TRUE) -> (w195:T3)
            n95 = call "Counter Presets.vi"("error in (no error)"=w203, "Number of triggers"=w199, "Counter (Def: T)"=enum16{"Invalid", "Counter B", "Counter T"}."Counter T" ("i (0) 2"), "VISA resource name"=w204) -> ("error out"=w209:errorcluster, "VISA resource name out"=w206:refnum<visa-resource-name>)  [unwired: 6 out]
            n96 = call "Query Counter presets.vi"("error in (no error)"=w209, "Counter (Def: T)"=enum16{"Invalid", "Counter B", "Counter T"}."Counter T" ("i (0)"), "VISA resource name"=w206) -> ("error out"=w208:errorcluster, "Number of triggers"=w210:dbl, "VISA resource name out"=w207:refnum<visa-resource-name>)  [unwired: 6 out]
            n97 = local write "Actual"(w210) -> ()
          }
          event "Set # of Triggers": Value Change {
            # "Frechem: Did not change"
            n98 = event-data() -> ()  [unwired: 7 out]
            n99 = local read "Target"() -> (w221:dbl)
            n100 = call "Set Counter Input.vi"("error in (no error)"=w223, "Input (def: 10 MHz)"=enum16{"10 MHz", "INPUT 1", "INPUT 2", "TRIG"}."TRIG" ("n (0.000000)"), "Counter (def: A)"=enum16{"Counter A", "Counter B", "Counter T"}."Counter T" ("i (0) 2"), "VISA resource name"=w224) -> ("error out"=w225:errorcluster, "VISA resource name out"=w226:refnum<visa-resource-name>)  [unwired: 6 out]
            n101 = call "round to one sig fig.vi"("input number"=w221) -> ("rounded to 1 sig fig"=w219:dbl)
            n102 = call "Counter Presets.vi"("error in (no error)"=w225, "Number of triggers"=w219, "Counter (Def: T)"=enum16{"Invalid", "Counter B", "Counter T"}."Counter T" ("i (0) 2"), "VISA resource name"=w226) -> ("error out"=w229:errorcluster, "VISA resource name out"=w228:refnum<visa-resource-name>)  [unwired: 6 out]
            n103 = call "Query Counter presets.vi"("error in (no error)"=w229, "Counter (Def: T)"=enum16{"Invalid", "Counter B", "Counter T"}."Counter T" ("i (0)"), "VISA resource name"=w228) -> ("error out"=w230:errorcluster, "Number of triggers"=w218:dbl, "VISA resource name out"=w231:refnum<visa-resource-name>)  [unwired: 6 out]
            "Actual" <- w218
            n104 = local read "Actual"() -> (w213:dbl[unit])
            n105 = Divide(x=w221, y=w213) -> (x/y=w220:dbl[unit])
            n106 = Divide(x=w218, y=w213) -> (x/y=w215:dbl[unit])
            n107 = local write "Actual"(w215) -> ()
            n108 = local write "Target"(w220) -> ()
            n109 = Bundle By Name(cluster=w217, "Count Time"=w215, "Trigger Frequency"=w213, "Trigger External?"=TRUE) -> (w216:T3)
          }
          event "Start Unmonitored Scan": Value Change {
            # "This presses the start button on the front panel to start a scan. The original method was only ideal\nfor a single period scan and it would cause the data to be read out very slowly. The current way \nstarts a scan and the user has to be aware that data can't be written from buffer until the scan ends.\nI am working on a way to prevent the save button from being pressed until scan is over without \ngetting rid of the functionality of the stop button.\n\nThis event is unused but I left it in case you want to use the start and stop buttons without the monitoring."
            n110 = event-data() -> ()  [unwired: 7 out]
            n111 = flat-sequence {
              tunnel: w239 -> [w250]
              tunnel: w237 -> [w249]
              tunnel: w245 -> [w247]
              tunnel: [w246] -> w236
              tunnel: [w248] -> w235
              tunnel: [w250] -> w234
              tunnel: [w256] -> w244
              tunnel: [w254] -> w242
              tunnel: [w253] -> w240
              tunnel: w236 -> [w257]
              tunnel: w235 -> [w255]
              tunnel: w234 -> [w253]
              tunnel: [w258] -> w243
              tunnel: w244 -> [w258]
              tunnel: w242 -> [w259]
              tunnel: [w259] -> w241
              tunnel: [w260] -> w238
              tunnel: w240 -> [w260]
              frame #0 {
                n112 = call "Reset Counters.vi"("error in (no error)"=w247, "VISA resource name"=w249) -> ("error out"=w246:errorcluster, "VISA resource name out"=w248:refnum<visa-resource-name>)  [unwired: 8 in]
              }
              frame #1 {
                n113 = Get Date/Time In Seconds() -> (seconds since 1Jan1904=w252:timestamp)
                "Scan Start Time" <- w252
                n114 = Format Date/Time String(seconds (now)=w252) -> (date/time string=w251:string)  [unwired: 2 in]
                n115 = Build Array(w251) -> ()  [unwired: 1 out]
                n116 = call "Start button.vi"("error in (no error)"=w257, "VISA resource name"=w255) -> ("error out"=w256:errorcluster, "VISA resource name out"=w254:refnum<visa-resource-name>)  [unwired: 8 in]
              }
              frame #2 {
                n117 = local write "Start Unmonitored Scan"(FALSE ("Read Channels")) -> ()
              }
            }
          }
          event "Monitor": Value Change {
            # "This simply monitors the counts on the hardware front panel\nusing the \"XA\" and \"XB\" commands. Added by Frechem."
            n118 = event-data() -> ()  [unwired: 7 out]
            n119 = while {
              tunnel: w263 -> [w270]
              tunnel: [w269] -> w262
              tunnel: w264 -> [w271]
              tunnel: [w273] -> w266
              tunnel: w265 -> [w272]
              tunnel: [w274] -> w267
              stop <- "Monitor" stop-if-true
              n120 = flat-sequence {
                tunnel: w271 -> [w280]
                tunnel: [w280] -> w277
                tunnel: w272 -> [w279]
                tunnel: [w279] -> w276
                tunnel: w270 -> [w278]
                tunnel: [w278] -> w275
                tunnel: w277 -> [w284]
                tunnel: w276 -> [w283]
                tunnel: w275 -> [w282]
                tunnel: [w286] -> w273
                tunnel: [w285] -> w274
                tunnel: [w282] -> w269
                frame #0 {
                  n121 = Wait (ms)(milliseconds to wait=u32 50) -> ()  [unwired: 1 out]
                }
                frame #1 {
                  n122 = call "Query Count Display.vi"("error in (no error)"=w283, "Read B?"=FALSE, "VISA resource name"=w284) -> ("error out"=w291:errorcluster, "Counts"=→"Counter A":dbl, "VISA resource name out"=w289:refnum<visa-resource-name>)  [unwired: 6 in]
                  n123 = call "Query Count Display.vi"("error in (no error)"=w291, "Read B?"=TRUE, "VISA resource name"=w289) -> ("error out"=w285:errorcluster, "Counts"=→"Counter B":dbl, "VISA resource name out"=w286:refnum<visa-resource-name>)  [unwired: 6 in]
                }
              }
            }
          }
          event "Stop Unmonitored Scan": Value Change {
            # "This allows you to stop the scan at any point during the scan. \nIt simply presses the stop button on the front panel.\n\nThis is not in use as I combined start, monitor and stop. But, \nI left it in case someone wants to not use monitoring."
            n124 = event-data() -> ()  [unwired: 7 out]
            n125 = flat-sequence {
              tunnel: w297 -> [w303]
              tunnel: w295 -> [w302]
              tunnel: [w300] -> w299
              tunnel: [w302] -> w298
              tunnel: w296 -> [w304]
              tunnel: [w301] -> w294
              tunnel: [w306] -> w293
              tunnel: [w307] -> _
              tunnel: w299 -> [w307]
              tunnel: w298 -> [w306]
              frame #0 {
                n126 = call "Stop button.vi"("error in (no error)"=w303, "VISA resource name"=w304) -> ("error out"=w300:errorcluster, "VISA resource name out"=w301:refnum<visa-resource-name>)  [unwired: 8 in]
              }
              frame #1 {
                n127 = local write "Stop Unmonitored Scan"(FALSE ("Read Channels")) -> ()
              }
            }
          }
          event "Set Gate Delays": Value Change {
            # "Frechem: Did not change"
            n128 = event-data() -> ()  [unwired: 2 out]
            n129 = local read "Actual"() -> (w330:dbl[unit])
            n130 = local read "Actual"() -> (w329:dbl[unit])
            n131 = Divide(x=w330, y=2) -> (x/y=w310:dbl[unit])
            n132 = Divide(x=w329, y=2) -> (x/y=w311:dbl[unit])
            n133 = Subtract(x=w309, y=w310) -> (x-y=w326:dbl[unit])
            n134 = Subtract(x=w308, y=w311) -> (x-y=w324:dbl[unit])
            n135 = Select "T = referenced to middle\nF = reference to start"(t=w326, s="Start / Middle", f=w309) -> (s? t:f=w323:dbl[unit])
            n136 = Select(t=w324, s="Start / Middle", f=w308) -> (s? t:f=w325:dbl[unit])
            n137 = call "Set both gates.vi"("Error In"=w335, "VISA resource name"=w334, "Set Delay?"=TRUE, "gatedelayoffsetB"=w325, "gatedelayoffsetA"=w323) -> ("Error Out"=w320:errorcluster, "VISA resource name out"=w322:refnum<visa-resource-name>)  [unwired: 3 in, 2 out]
            n138 = call "Read both gates.vi"("error in (no error)"=w320, "VISA resource name"=w322) -> ("Gate B Delay"=w316:dbl[unit], "Gate A Delay"=w317:dbl[unit], "error out"=w319:errorcluster, "VISA resource name out"=w321:refnum<visa-resource-name>)  [unwired: 6 out]
            n139 = Add(x=w317, y=w310) -> (x+y=w315:dbl[unit])
            n140 = Add(x=w316, y=w311) -> (x+y=w314:dbl[unit])
            n141 = Select "T = referenced to middle\nF = reference to start"(t=w315, s="Start / Middle", f=w317) -> (s? t:f=w313:dbl[unit])
            n142 = Select(t=w314, s="Start / Middle", f=w316) -> (s? t:f=w312:dbl[unit])
            n143 = local write "Actual"(w312) -> ()
            n144 = local write "Actual"(w313) -> ()
            n145 = Bundle By Name(cluster=w333, "Gate A Delay"=w317, "Gate B Delay"=w316) -> (w332:T3)
          }
          event "Set Gate Widths": Value Change {
            # "Frechem: Did not change"
            n146 = event-data() -> ()  [unwired: 2 out]
            n147 = local read "Actual"() -> (w349:dbl[unit])
            n148 = local read "Gate Width: Time / Percent"() -> (w343:bool)
            n149 = call "gate percent to width.vi"("Trigger Freq"=w349, "Gate %"="Target") -> ("Gate width"=w345:dbl[unit])  [unwired: 1 out]
            n150 = call "gate percent to width.vi"("Trigger Freq"=w349, "Gate %"="Target") -> ("Gate width"=w344:dbl[unit])  [unwired: 1 out]
            n151 = Select(t=w345, s=w343, f=w336) -> (s? t:f=w346:dbl[unit])
            n152 = Select(t=w344, s=w343, f=w337) -> (s? t:f=w342:dbl[unit])
            n153 = call "Set both gates.vi"("Error In"=w354, "VISA resource name"=w355, "Set Width?"=TRUE, "Gate B Width"=w342, "Gate A Width"=w346) -> ("Error Out"=w358:errorcluster, "VISA resource name out"=w357:refnum<visa-resource-name>)  [unwired: 3 in, 2 out]
            n154 = call "Read both gates.vi"("error in (no error)"=w358, "VISA resource name"=w357) -> ("Gate B Width"=w338:dbl[unit], "Gate A Width"=w339:dbl[unit], "error out"=w352:errorcluster, "VISA resource name out"=w353:refnum<visa-resource-name>)  [unwired: 6 out]
            n155 = local write "Actual"(w339) -> ()
            n156 = local write "Actual"(w338) -> ()
            n157 = call "gate width to percent.vi"("Trigger Freq"=w349, "Gate width"=w339) -> ("Gate %"=w350:dbl)  [unwired: 1 out]
            n158 = call "gate width to percent.vi"("Trigger Freq"=w349, "Gate width"=w338) -> ("Gate %"=w351:dbl)  [unwired: 1 out]
            n159 = local write "Actual"(w350) -> ()
            n160 = local write "Actual"(w351) -> ()
            n161 = Bundle By Name(cluster=w341, "Gate A Width"=w339, "Gate B Width"=w338) -> (w340:T3)
          }
          event "Set Gate Mode": Value Change {
            # "Frechem: Did not change"
            n162 = event-data() -> ()  [unwired: 7 out]
            n163 = local write "Actual"(w359) -> ()
            n164 = local write "Actual"(w360) -> ()
            n165 = Bundle By Name(cluster=w362, "Gate A Mode"=w359, "Gate B Mode"=w360) -> (w361:T3)
            n166 = call "Set gate mode.vi"("error in (no error)"=w367, "Mode (def: CW)"=w359, "Gate (def: A)"=enum16{"Gate A", "Gate B"}."Gate A" ("i (0)"), "VISA resource name"=w368) -> ("error out"=w366:errorcluster, "VISA resource name out"=w365:refnum<visa-resource-name>)  [unwired: 6 out]
            n167 = call "Set gate mode.vi"("error in (no error)"=w366, "Mode (def: CW)"=w360, "Gate (def: A)"=enum16{"Gate A", "Gate B"}."Gate B" ("i (0)"), "VISA resource name"=w365) -> ("error out"=w364:errorcluster, "VISA resource name out"=w363:refnum<visa-resource-name>)  [unwired: 6 out]
          }
          event "Internal / External", "# Triggers vs Freq/Time": Value Change {
            # "Frechem: Did not change"
            n168 = event-data() -> ()  [unwired: 2 out]
            n169 = property on="Update visible/hidden" class="Bool (strict)"("Val(Sgnl)"=TRUE ("Value (Signaling)")) -> ()  [unwired: 2 in, 2 out]
          }
          event "Gate Width: Time / Percent": Value Change {
            # "Frechem: Did not change"
            # "Changes the gate widths to percents and updates values.\n\"Current\" is the value last read from the device."
            n170 = event-data() -> ("NewVal"=w379:bool)  [unwired: 6 out]
            n171 = local read "Actual"() -> (w380:dbl[unit])
            n172 = property on="Update visible/hidden" class="Bool (strict)"("Val(Sgnl)"=TRUE ("Value (Signaling)")) -> ()  [unwired: 2 in, 2 out]
            n173 = case shown="True" w379 {
              tunnel: w380 -> [w385 w401]
              tunnel: [w382 w392] -> w376
              tunnel: w375 -> [w382 w392]
              frame False {
                n174 = local read "Actual"() -> (w388:dbl)
                n175 = local read "Actual"() -> (w389:dbl)
                n176 = local read "Target"() -> (w383:dbl)
                n177 = local read "Target"() -> (w384:dbl)
                n178 = call "gate percent to width.vi"("Trigger Freq"=w385, "Gate %"=w388) -> ("Gate width"=w386:dbl[unit])  [unwired: 1 out]
                n179 = call "gate percent to width.vi"("Trigger Freq"=w385, "Gate %"=w389) -> ("Gate width"=w387:dbl[unit])  [unwired: 1 out]
                n180 = call "gate percent to width.vi"("Trigger Freq"=w385, "Gate %"=w383) -> ("Gate width"=w391:dbl[unit])  [unwired: 1 out]
                n181 = call "gate percent to width.vi"("Trigger Freq"=w385, "Gate %"=w384) -> ("Gate width"=w390:dbl[unit])  [unwired: 1 out]
                n182 = local write "Actual"(w386) -> ()
                n183 = local write "Actual"(w387) -> ()
                n184 = local write "Target"(w391) -> ()
                n185 = local write "Target"(w390) -> ()
              }
              frame True {
                n186 = local read "Target"() -> (w400:dbl[unit])
                n187 = local read "Target"() -> (w398:dbl[unit])
                n188 = local read "Actual"() -> (w396:dbl[unit])
                n189 = local read "Actual"() -> (w394:dbl[unit])
                n190 = call "gate width to percent.vi"("Trigger Freq"=w401, "Gate width"=w400) -> ("Gate %"=w399:dbl)  [unwired: 1 out]
                n191 = call "gate width to percent.vi"("Trigger Freq"=w401, "Gate width"=w398) -> ("Gate %"=w397:dbl)  [unwired: 1 out]
                n192 = call "gate width to percent.vi"("Trigger Freq"=w401, "Gate width"=w396) -> ("Gate %"=w395:dbl)  [unwired: 1 out]
                n193 = call "gate width to percent.vi"("Trigger Freq"=w401, "Gate width"=w394) -> ("Gate %"=w393:dbl)  [unwired: 1 out]
                n194 = local write "Target"(w399) -> ()
                n195 = local write "Target"(w397) -> ()
                n196 = local write "Actual"(w395) -> ()
                n197 = local write "Actual"(w393) -> ()
              }
            }
          }
          event "Start / Middle": Value Change {
            # "Frechem: Did not change"
            # "Updates the gate widths depending on when it is set."
            n198 = event-data() -> ("NewVal"=w405:bool)  [unwired: 6 out]
            n199 = case shown="False" w405 {
              frame False {
                n200 = local read "Actual"() -> (w416:dbl[unit])
                n201 = local read "Actual"() -> (w419:dbl[unit])
                n202 = Divide(x=w416, y=2) -> (x/y=w410:dbl[unit])
                n203 = Divide(x=w419, y=2) -> (x/y=w415:dbl[unit])
                n204 = local read "Actual"() -> (w407:dbl[unit])
                n205 = local read "Target"() -> (w409:dbl[unit])
                n206 = local read "Actual"() -> (w412:dbl[unit])
                n207 = local read "Target"() -> (w414:dbl[unit])
                n208 = Subtract(x=w407, y=w410) -> (x-y=w406:dbl[unit])
                n209 = Subtract(x=w409, y=w410) -> (x-y=w408:dbl[unit])
                n210 = Subtract(x=w412, y=w415) -> (x-y=w411:dbl[unit])
                n211 = Subtract(x=w414, y=w415) -> (x-y=w413:dbl[unit])
                n212 = local write "Actual"(w406) -> ()
                n213 = local write "Target"(w408) -> ()
                n214 = local write "Actual"(w411) -> ()
                n215 = local write "Target"(w413) -> ()
              }
              frame True {
                n216 = local read "Actual"() -> (w433:dbl[unit])
                n217 = local read "Actual"() -> (w430:dbl[unit])
                n218 = Divide(x=w433, y=2) -> (x/y=w429:dbl[unit])
                n219 = Divide(x=w430, y=2) -> (x/y=w424:dbl[unit])
                n220 = local read "Actual"() -> (w426:dbl[unit])
                n221 = local read "Target"() -> (w428:dbl[unit])
                n222 = local read "Actual"() -> (w421:dbl[unit])
                n223 = local read "Target"() -> (w423:dbl[unit])
                n224 = Add(x=w426, y=w429) -> (x+y=w425:dbl[unit])
                n225 = Add(x=w428, y=w429) -> (x+y=w427:dbl[unit])
                n226 = Add(x=w421, y=w424) -> (x+y=w420:dbl[unit])
                n227 = Add(x=w423, y=w424) -> (x+y=w422:dbl[unit])
                n228 = local write "Actual"(w425) -> ()
                n229 = local write "Target"(w427) -> ()
                n230 = local write "Actual"(w420) -> ()
                n231 = local write "Target"(w422) -> ()
              }
            }
          }
          event "Update visible/hidden": Value Change {
            n232 = event-data() -> ()  [unwired: 7 out]
            n233 = local write "Update visible/hidden"(FALSE ("Update visiible/hidden")) -> ()
            n234 = flat-sequence {
              frame #0 {
                n235 = property on="Actual" class="DigNum (strict)"("Visible"="Gate Width: Time / Percent") -> ()  [unwired: 2 in, 2 out]
                n236 = property on="Actual" class="DigNum (strict)"("Visible"="Gate Width: Time / Percent") -> ()  [unwired: 2 in, 2 out]
                n237 = property on="Target" class="DigNum (strict)"("Visible"="Gate Width: Time / Percent") -> ()  [unwired: 2 in, 2 out]
                n238 = Not(x="Gate Width: Time / Percent") -> (.not. x?=w439:bool)
                n239 = property on="Target" class="DigNum (strict)"("Visible"=w439) -> ()  [unwired: 2 in, 2 out]
                n240 = property on="Actual" class="DigNum (strict)"("Visible"=w439) -> ()  [unwired: 2 in, 2 out]
                n241 = property on="Actual" class="DigNum (strict)"("Visible"=w439) -> ()  [unwired: 2 in, 2 out]
                n242 = property on="Target" class="DigNum (strict)"("Visible"=w439) -> ()  [unwired: 2 in, 2 out]
                n243 = property on="Target" class="DigNum (strict)"("Visible"="Gate Width: Time / Percent") -> ()  [unwired: 2 in, 2 out]
              }
              frame #1 {
                # "Frechem: Did not change"
                n244 = local read "# Triggers vs Freq/Time"() -> (w441:bool)
                n245 = local read "Internal / External"() -> (w442:bool)
                n246 = property on="# Triggers vs Freq/Time" class="Bool (strict)"("Visible"=w442) -> ()  [unwired: 2 in, 2 out]
                n247 = Not(x=w441) -> (.not. x?=w443:bool)
                n248 = And(x=w442, y=w441) -> (x .and. y?=w445:bool)
                n249 = Not(x=w442) -> (.not. x?=w440:bool)
                n250 = property on="Set Count Time" class="Bool"("Visible"=w440) -> ()  [unwired: 2 in, 2 out]
                n251 = property on="Target" class="DigNum (strict)"("Visible"=w445) -> ()  [unwired: 2 in, 2 out]
                n252 = property on="Actual" class="DigNum (strict)"("Visible"=w445) -> ()  [unwired: 2 in, 2 out]
                n253 = Or(x=w440, y=w441) -> (x .or. y?=w446:bool)
                n254 = And(x=w442, y=w443) -> (x .and. y?=w444:bool)
                n255 = property on="Target" class="DigNum (strict)"("Visible"=w444) -> ()  [unwired: 2 in, 2 out]
                n256 = property on="Actual" class="DigNum (strict)"("Visible"=w444) -> ()  [unwired: 2 in, 2 out]
                n257 = property on="Actual" class="DigNum (strict)"("Visible"=w446) -> ()  [unwired: 2 in, 2 out]
                n258 = property on="Target" class="DigNum (strict)"("Visible"=w446) -> ()  [unwired: 2 in, 2 out]
                n259 = property on="Set Time & Freq." class="Bool"("Visible"=w445) -> ()  [unwired: 2 in, 2 out]
                n260 = property on="Set # of Triggers" class="Bool"("Visible"=w444) -> ()  [unwired: 2 in, 2 out]
              }
            }
          }
          event "Set # Periods": Value Change {
            # "This allows you to update the number of periods to be taken while the device is running\nwithout being reinitialized."
            n261 = event-data() -> ()  [unwired: 2 out]
            n262 = call "Set Num Periods.vi"("# of periods"=w447, "Set # Periods"="Set # Periods", "Error In"=w449, "VISA resource name"=w450) -> ("Error Out"=w456:errorcluster, "VISA resource name out"=w455:refnum<visa-resource-name>)  [unwired: 6 in]
            n263 = call "Get Number Periods.vi"("error in (no error)"=w456, "VISA resource name"=w455) -> ("error out"=w451:errorcluster, "# Periods"=→"Actual":dbl, "VISA resource name out"=w452:refnum<visa-resource-name>)  [unwired: 7 in]
          }
          event "Set Dwell Time": Value Change {
            # "This allows you to update the dwell time\nwithout reinitialization."
            n264 = event-data() -> ()  [unwired: 7 out]
            n265 = call "Set Dwell Time.vi"("Error In"=w465, "Dwell time"=w463, "Set # Periods"="Set Dwell Time", "VISA resource name"=w466) -> ("Error Out"=w461:errorcluster, "VISA resource name out"=w462:refnum<visa-resource-name>)  [unwired: 6 in]
            n266 = call "Get Dwell Time.vi"("error in (no error)"=w461, "VISA resource name"=w462) -> ("error out"=w458:errorcluster, "output"=→"Actual":dbl[unit], "VISA resource name out"=w459:refnum<visa-resource-name>)  [unwired: 7 in]
          }
          event "Read Buffer Data": Value Change {
            # "Read data from buffer courtesy of Paul Henning on the\nNational Instruments forum."
            n267 = event-data() -> ()  [unwired: 7 out]
            n268 = local write "Read Buffer Data"(FALSE ("Read Buffer Data")) -> ()
            n269 = flat-sequence {
              tunnel: w477 -> [w490]
              tunnel: w479 -> [w489]
              tunnel: w481 -> [w488]
              tunnel: w483 -> [w487]
              tunnel: [w484] -> w475
              tunnel: [w485] -> w474
              tunnel: [w489] -> w473
              tunnel: [w490] -> w472
              tunnel: [w486] -> w471
              tunnel: w476 -> [w491]
              tunnel: w475 -> [w498]
              tunnel: w474 -> [w496]
              tunnel: w473 -> [w494]
              tunnel: w472 -> [w492]
              tunnel: [w497] -> w470
              tunnel: [w495] -> w469
              tunnel: [w493] -> w468
              tunnel: [w570] -> w478
              tunnel: [w566] -> w480
              tunnel: [w567] -> w482
              tunnel: w470 -> [w568]
              tunnel: w469 -> [w569]
              tunnel: w468 -> [w570]
              frame #0 {
                n270 = call "Query Status Byte.vi"("error in (no error)"=w487, "VISA resource name"=w488) -> ("error out"=w484:errorcluster, "Status Register"=w486:T5, "VISA resource name out"=w485:refnum<visa-resource-name>)  [unwired: 7 in]
              }
              frame #1 {
                n271 = case shown="True" w491 {
                  tunnel: w498 -> [w499 w508]
                  tunnel: [w499 w507] -> w497
                  tunnel: w496 -> [w500 w506]
                  tunnel: [w500 w505] -> w495
                  tunnel: w494 -> [w501 w504]
                  tunnel: [w501 w503] -> w493
                  tunnel: w492 -> [_ w502]
                  frame False {
                  }
                  frame True {
                    n272 = flat-sequence {
                      tunnel: [w521] -> w507
                      tunnel: [w522] -> w505
                      tunnel: [w523] -> w503
                      tunnel: w502 -> [w524]
                      tunnel: w508 -> [w521]
                      tunnel: w506 -> [w522]
                      tunnel: w504 -> [w523]
                      frame #0 {
                        n273 = Number To Decimal String(number="GPIB Address") -> (decimal integer string=w530:string)  [unwired: 1 in]
                        n274 = call "Read Data.vi"("Channel Number"=0, "GPIB Address"=w530, "Number of Datapoints"=w524) -> ("Data"=w525:i32[])
                        n275 = call "Read Data.vi"("Channel Number"=1, "GPIB Address"=w530, "Number of Datapoints"=w524) -> ("Data"=w526:i32[])
                        n276 = call "Convert to Dynamic Data"("Array"=w525) -> ("Dynamic Data Type"=w512:dynamicdata)  [unwired: 3 in]
                        n277 = call "Convert to Dynamic Data2"("Array"=w526) -> ("Dynamic Data Type"=w513:dynamicdata)  [unwired: 3 in]
                        n278 = xnode "Set Dynamic Data Attributes"("Signals In"=w512, "Signal Index"=0, "Signal Name"="Counter A", "Unit"="Counts") -> ("Signals Out"=w510:dynamicdata)  [unwired: 1 in, 1 out]
                        n279 = xnode "Set Dynamic Data Attributes"("Signals In"=w513, "Signal Index"=1, "Signal Name"="Counter B", "Unit"="Counts") -> ("Signals Out"=w509:dynamicdata)  [unwired: 1 in, 1 out]
                        n280 = Merge Signals(w510, w509) -> (w511:dynamicdata)
                        n281 = call "Write LabVIEW Measurement File"("Signals"=w511, "Enable"=TRUE) -> ("Filename Out"=→"Filename Out":path)  [unwired: 15 in, 2 out]
                      }
                    }
                  }
                }
              }
              frame #2 {
                n282 = call "Reset Counters.vi"("error in (no error)"=w568, "VISA resource name"=w569) -> ("error out"=w567:errorcluster, "VISA resource name out"=w566:refnum<visa-resource-name>)  [unwired: 8 in]
              }
            }
          }
          event "Start Scan": Value Change {
            # "This allows you to start and stop a scan with the counts being polled from the hardware front display. \nI tried to implement it other ways but my LabVIEW knowledge limited how I could approach it."
            n283 = event-data() -> ()  [unwired: 7 out]
            n284 = flat-sequence {
              tunnel: w577 -> [w643]
              tunnel: w576 -> [w642]
              tunnel: w575 -> [w640]
              tunnel: [w639] -> w586
              tunnel: [w641] -> w585
              tunnel: [w643] -> w584
              tunnel: [w649] -> w583
              tunnel: [w647] -> w582
              tunnel: [w646] -> w581
              tunnel: w586 -> [w650]
              tunnel: w585 -> [w648]
              tunnel: w584 -> [w646]
              tunnel: [w652] -> w579
              tunnel: w583 -> [w652]
              tunnel: w582 -> [w651]
              tunnel: [w653] -> w578
              tunnel: w581 -> [w653]
              tunnel: [w651] -> w580
              frame #0 {
                n285 = call "Reset Counters.vi"("error in (no error)"=w640, "VISA resource name"=w642) -> ("error out"=w639:errorcluster, "VISA resource name out"=w641:refnum<visa-resource-name>)  [unwired: 8 in]
              }
              frame #1 {
                n286 = call "Start button.vi"("error in (no error)"=w650, "VISA resource name"=w648) -> ("error out"=w649:errorcluster, "VISA resource name out"=w647:refnum<visa-resource-name>)  [unwired: 8 in]
                n287 = Get Date/Time In Seconds() -> (seconds since 1Jan1904=w645:timestamp)
                "Scan Start Time" <- w645
                n288 = Format Date/Time String(seconds (now)=w645) -> (date/time string=w644:string)  [unwired: 2 in]
                n289 = Build Array(w644) -> ()  [unwired: 1 out]
              }
              frame #2 {
                n290 = local write "Start Scan"(FALSE ("Read Channels")) -> ()
              }
            }
            n291 = while {
              tunnel: [w591] -> w573
              tunnel: w580 -> [w592]
              tunnel: [w594] -> w572
              tunnel: w579 -> [w593]
              tunnel: [w595] -> w574
              tunnel: w578 -> [w590]
              tunnel: [w587] -> w571
              stop <- w588 stop-if-true
              n292 = flat-sequence {
                tunnel: w592 -> [w604]
                tunnel: [w604] -> w600
                tunnel: w593 -> [w603]
                tunnel: [w603] -> w599
                tunnel: w590 -> [w602]
                tunnel: [w602] -> w589
                tunnel: ["Stop Scan"] -> w588
                tunnel: [w607] -> w598
                tunnel: [w606] -> w597
                tunnel: w600 -> [w610]
                tunnel: w599 -> [w609]
                tunnel: [w608] -> w596
                tunnel: w589 -> [w608]
                tunnel: [w619] -> w595
                tunnel: [w618] -> w594
                tunnel: w598 -> [w620]
                tunnel: w597 -> [w623]
                tunnel: w596 -> [w622]
                tunnel: [w621] -> w591
                tunnel: w588 -> [w624]
                tunnel: [w617] -> w587
                frame #0 {
                  n293 = Wait (ms)(milliseconds to wait=u32 5) -> ()  [unwired: 1 out]
                }
                frame #1 {
                  n294 = call "Query Count Display.vi"("error in (no error)"=w609, "Read B?"=FALSE, "VISA resource name"=w610) -> ("error out"=w615:errorcluster, "Counts"=→"Counter A":dbl, "VISA resource name out"=w613:refnum<visa-resource-name>)  [unwired: 6 in]
                  n295 = call "Query Count Display.vi"("error in (no error)"=w615, "Read B?"=TRUE, "VISA resource name"=w613) -> ("error out"=w606:errorcluster, "Counts"=→"Counter B":dbl, "VISA resource name out"=w607:refnum<visa-resource-name>)  [unwired: 6 in]
                }
                frame #2 {
                  n296 = case shown="True" w624 {
                    tunnel: w623 -> [w629 w636]
                    tunnel: w620 -> [w628 w637]
                    tunnel: w622 -> [w630 w638]
                    tunnel: [w630 w638] -> w621
                    tunnel: [w626 w631] -> w619
                    tunnel: [w627 w632] -> w618
                    tunnel: [w625 w633] -> w617
                    frame False {
                      n297 = call "Query Status Byte.vi"("error in (no error)"=w629, "VISA resource name"=w628) -> ("error out"=w626:errorcluster, "Status Register"=w625:T5, "VISA resource name out"=w627:refnum<visa-resource-name>)  [unwired: 7 in]
                    }
                    frame True {
                      n298 = call "Stop button.vi"("error in (no error)"=w636, "VISA resource name"=w637) -> ("error out"=w634:errorcluster, "VISA resource name out"=w635:refnum<visa-resource-name>)  [unwired: 8 in]
                      n299 = call "Query Status Byte.vi"("error in (no error)"=w634, "VISA resource name"=w635) -> ("error out"=w631:errorcluster, "Status Register"=w633:T5, "VISA resource name out"=w632:refnum<visa-resource-name>)  [unwired: 7 in]
                    }
                  }
                }
              }
            }
          }
        }
        n300 = Unbundle(w25) -> ("Data Ready"=w24:bool, "Scan Finished"=→"Scan Done":bool)  [unwired: 9 out]
        "Data Ready" <- w24
        n301 = feedback-in #1(w24) -> ()
        n302 = call <vilib>:"Simple Error Handler.vi"("error in (no error)"=w39) -> ("error out"=w38:errorcluster)  [unwired: 1 in, 7 out]
      }
    }
    frame #2 {
    }
  }
  "error out" <- w2
